vi "CALCULADORA SIRSA.vi"() -> ()   [LabVIEW 2018]
panel:
  in  "stop":bool
  out "RESULTADO":dbl
  in  "CALCULAR":bool
  in  "VALOR A CALCULAR":dbl
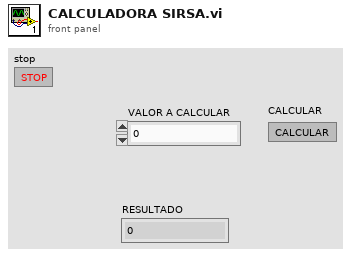
[diagram p1: front panel]
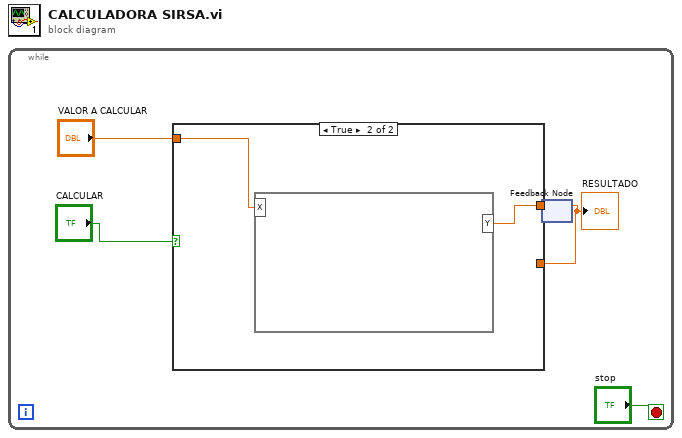
[diagram p0: block diagram]
diagram:
  n1 = while {
    stop <- "stop" stop-if-true
    n2 = feedback #1() -> (w1:dbl)  [unwired: 1 in]
    "RESULTADO" <- w1
    n3 = case shown="True" "CALCULAR" {
      tunnel: [w6 w8] -> w2
      tunnel: "VALOR A CALCULAR" -> [_ w7]
      tunnel: w1 -> [w6 _]
      frame False {
      }
      frame True {
        n4 = formula code=""("X"=w7) -> ("Y"=w8:dbl)
      }
    }
    n5 = feedback-in #1(w2) -> ()
  }
